vi "PlayWithLMSVector.vi"() -> ()   [LabVIEW 2014]
panel:
  out "dist":i32[](array[numeric])
  out "d(ang)":i32[](array[numeric])
  out "ang":dbl
  out "RY":dbl
  out "RX":dbl
  out "sim course":i8[][](array[numeric])
  in  "Robot Heading":dbl
  in  "Robot Long":dbl=81.2675 format="%#_8g"
  in  "Robot Lat":dbl=37.1526 format="%#_8g"
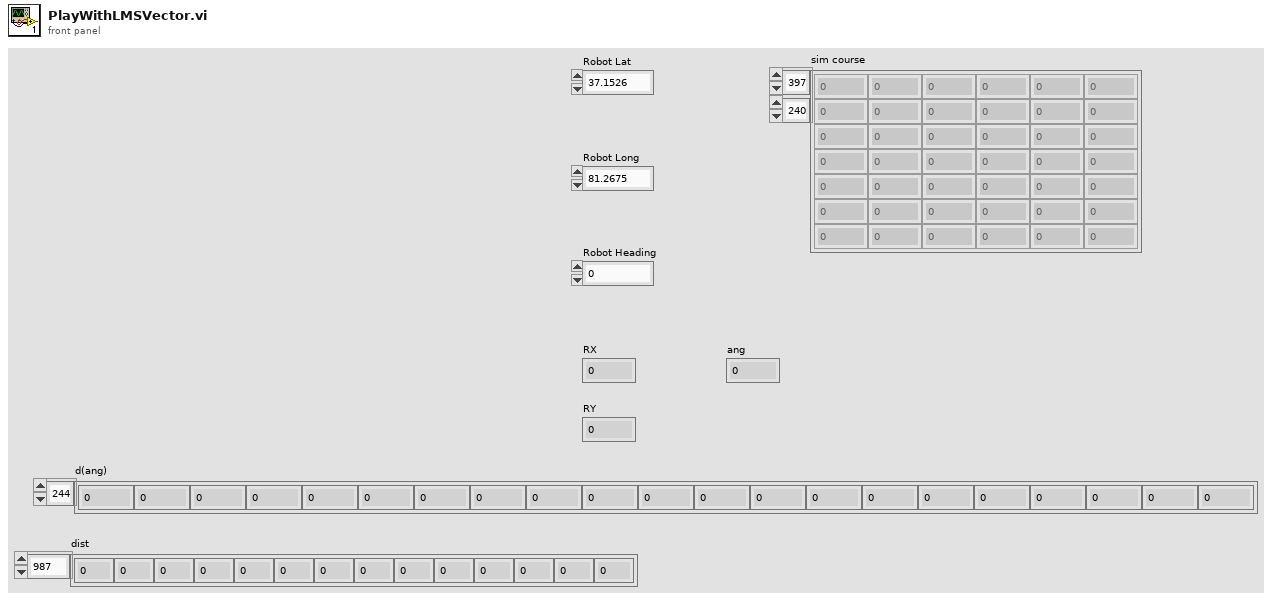
[diagram p1: front panel]
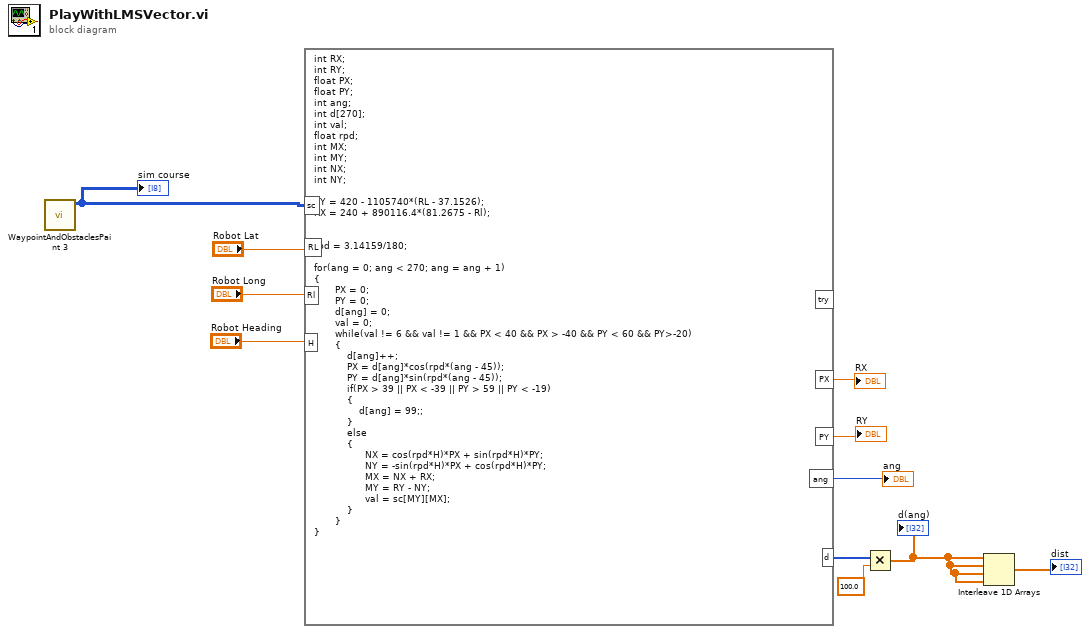
[diagram p0: block diagram]
diagram:
  n1 = call "WaypointAndObstaclesPaint 3.vi"() -> (3:w11:u8[][])  [unwired: 10 in, 1 out]
  "sim course" <- w11
  n2 = formula code="int RX;\nint RY;\nfloat PX;\nfloat PY;\nint ang;\nint d[270];\nint val;\nfloat rpd;\nint MX;\nint MY;\nint NX;\nint NY;\n\nRY = 420 - 1105740*(RL - 37.1526);\nRX = 240 + 890116.4*(81.2675 - Rl);\n\n\nrpd = 3.14159/180;\n\nfor(ang = 0; ang < 270; ang = ang + 1)\n{\n       PX = 0;\n       PY = 0;\n       d[ang] = 0;\n       val = 0;\n       while(val != 6 && val != 1 && PX < 40 && PX > -40 && PY < 60 && PY>-20) \n       {\n           d[ang]++;\n           PX = d[ang]*cos(rpd*(ang - 45));\n           PY = d[ang]*sin(rpd*(ang - 45));\n           if(PX > 39 || PX < -39 || PY > 59 || PY < -19)\n           {\n               d[ang] = 99;;\n           }\n           else\n           {\n                 NX = cos(rpd*H)*PX + sin(rpd*H)*PY;\n                 NY = -sin(rpd*H)*PX + cos(rpd*H)*PY;\n                 MX = NX + RX;\n                 MY = RY - NY;\n                 val = sc[MY][MX];\n           }\n       }\n}"("sc"=w11, "RL"="Robot Lat", "Rl"="Robot Long", "H"="Robot Heading") -> ("PX"=→"RX":dbl, "PY"=→"RY":dbl, "ang"=→"ang":i32, "d"=w1:i32[])  [unwired: 1 out]
  n3 = Multiply(x=w1, y=100.0) -> (x*y=w3:dbl[])
  "d(ang)" <- w3
  n4 = Interleave 1D Arrays(w3, w3, w3, w3) -> (→"dist":dbl[])
